vi "_Initialise Hardware Splash.vi"(8 "error in (no error)":errorcluster) -> (0 "error out":errorcluster, 2 "VISA Refnum out":refnum<visa-resource-name>, 3 "Enabled Hardware":T1)   [LabVIEW 2020]
uses:
  _Controls/Enabled Hardware.ctl
panel:
  in  "Enabled Hardware":T1=[{"Enable"=TRUE, "Status"=FALSE, "Device"="Confocal"}, {"Enable"=TRUE, "Status"=FALSE, "Device"="Pinhole"}, {"Enable"=TRUE, "Status"=FALSE, "Device"="Piezo"}, {"Enable"=TRUE, "Status"=FALSE, "Device"="iFlex"}, {"Enable"=TRUE, "Status"=FALSE, "Device"="Manlight"}, {"Enable"=TRUE, "Status"=FALSE, "Device"="SLM"}, {"Enable"=FALSE, "Status"=FALSE, "Device"="Camera"}]
  in  "Review":bool
  in  "Scan For Missing":bool
  out "SLM":bool
  out "iFlex":bool
  out "Manlight":bool
  out "Pinhole":bool
  out "PIFOC":bool
  out "Confocal":bool
  in  "animation":u16(ring)
  out "Status":string
  in  "Start":bool
  # "TweezerTron"
  # "Scanning for system hardware."
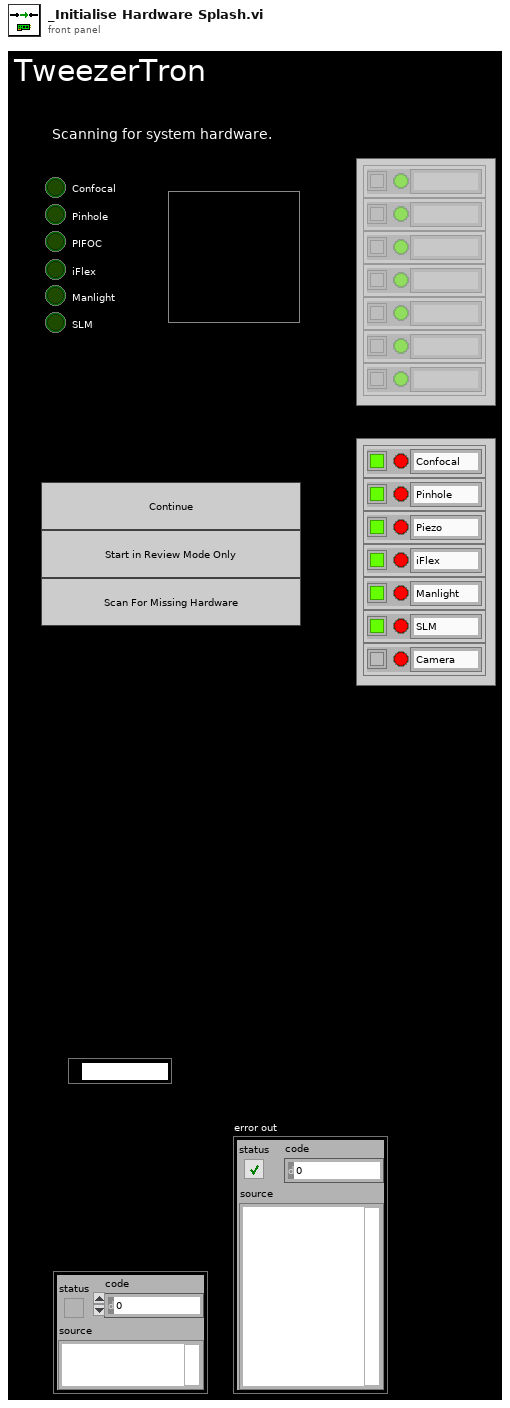
[diagram p1: front panel]
types:
  T1 = typedef "Enabled Hardware.ctl" = cluster{"Enable":bool, "Status":bool, "Device":string}[]
  T2 = typedef "Enabled Hardware.ctl" = cluster{"Confocal":cluster{"Enable":bool, "Status":bool}, "Pinhole":cluster{"Enable":bool, "Status":bool}, "Piezo":cluster{"Enable":bool, "Status":bool}, "iFlex":cluster{"Enable":bool, "Status":bool}, "SLM":cluster{"Enable":bool, "Status":bool}, "Manlight":cluster{"Enable":bool, "Status":bool}}
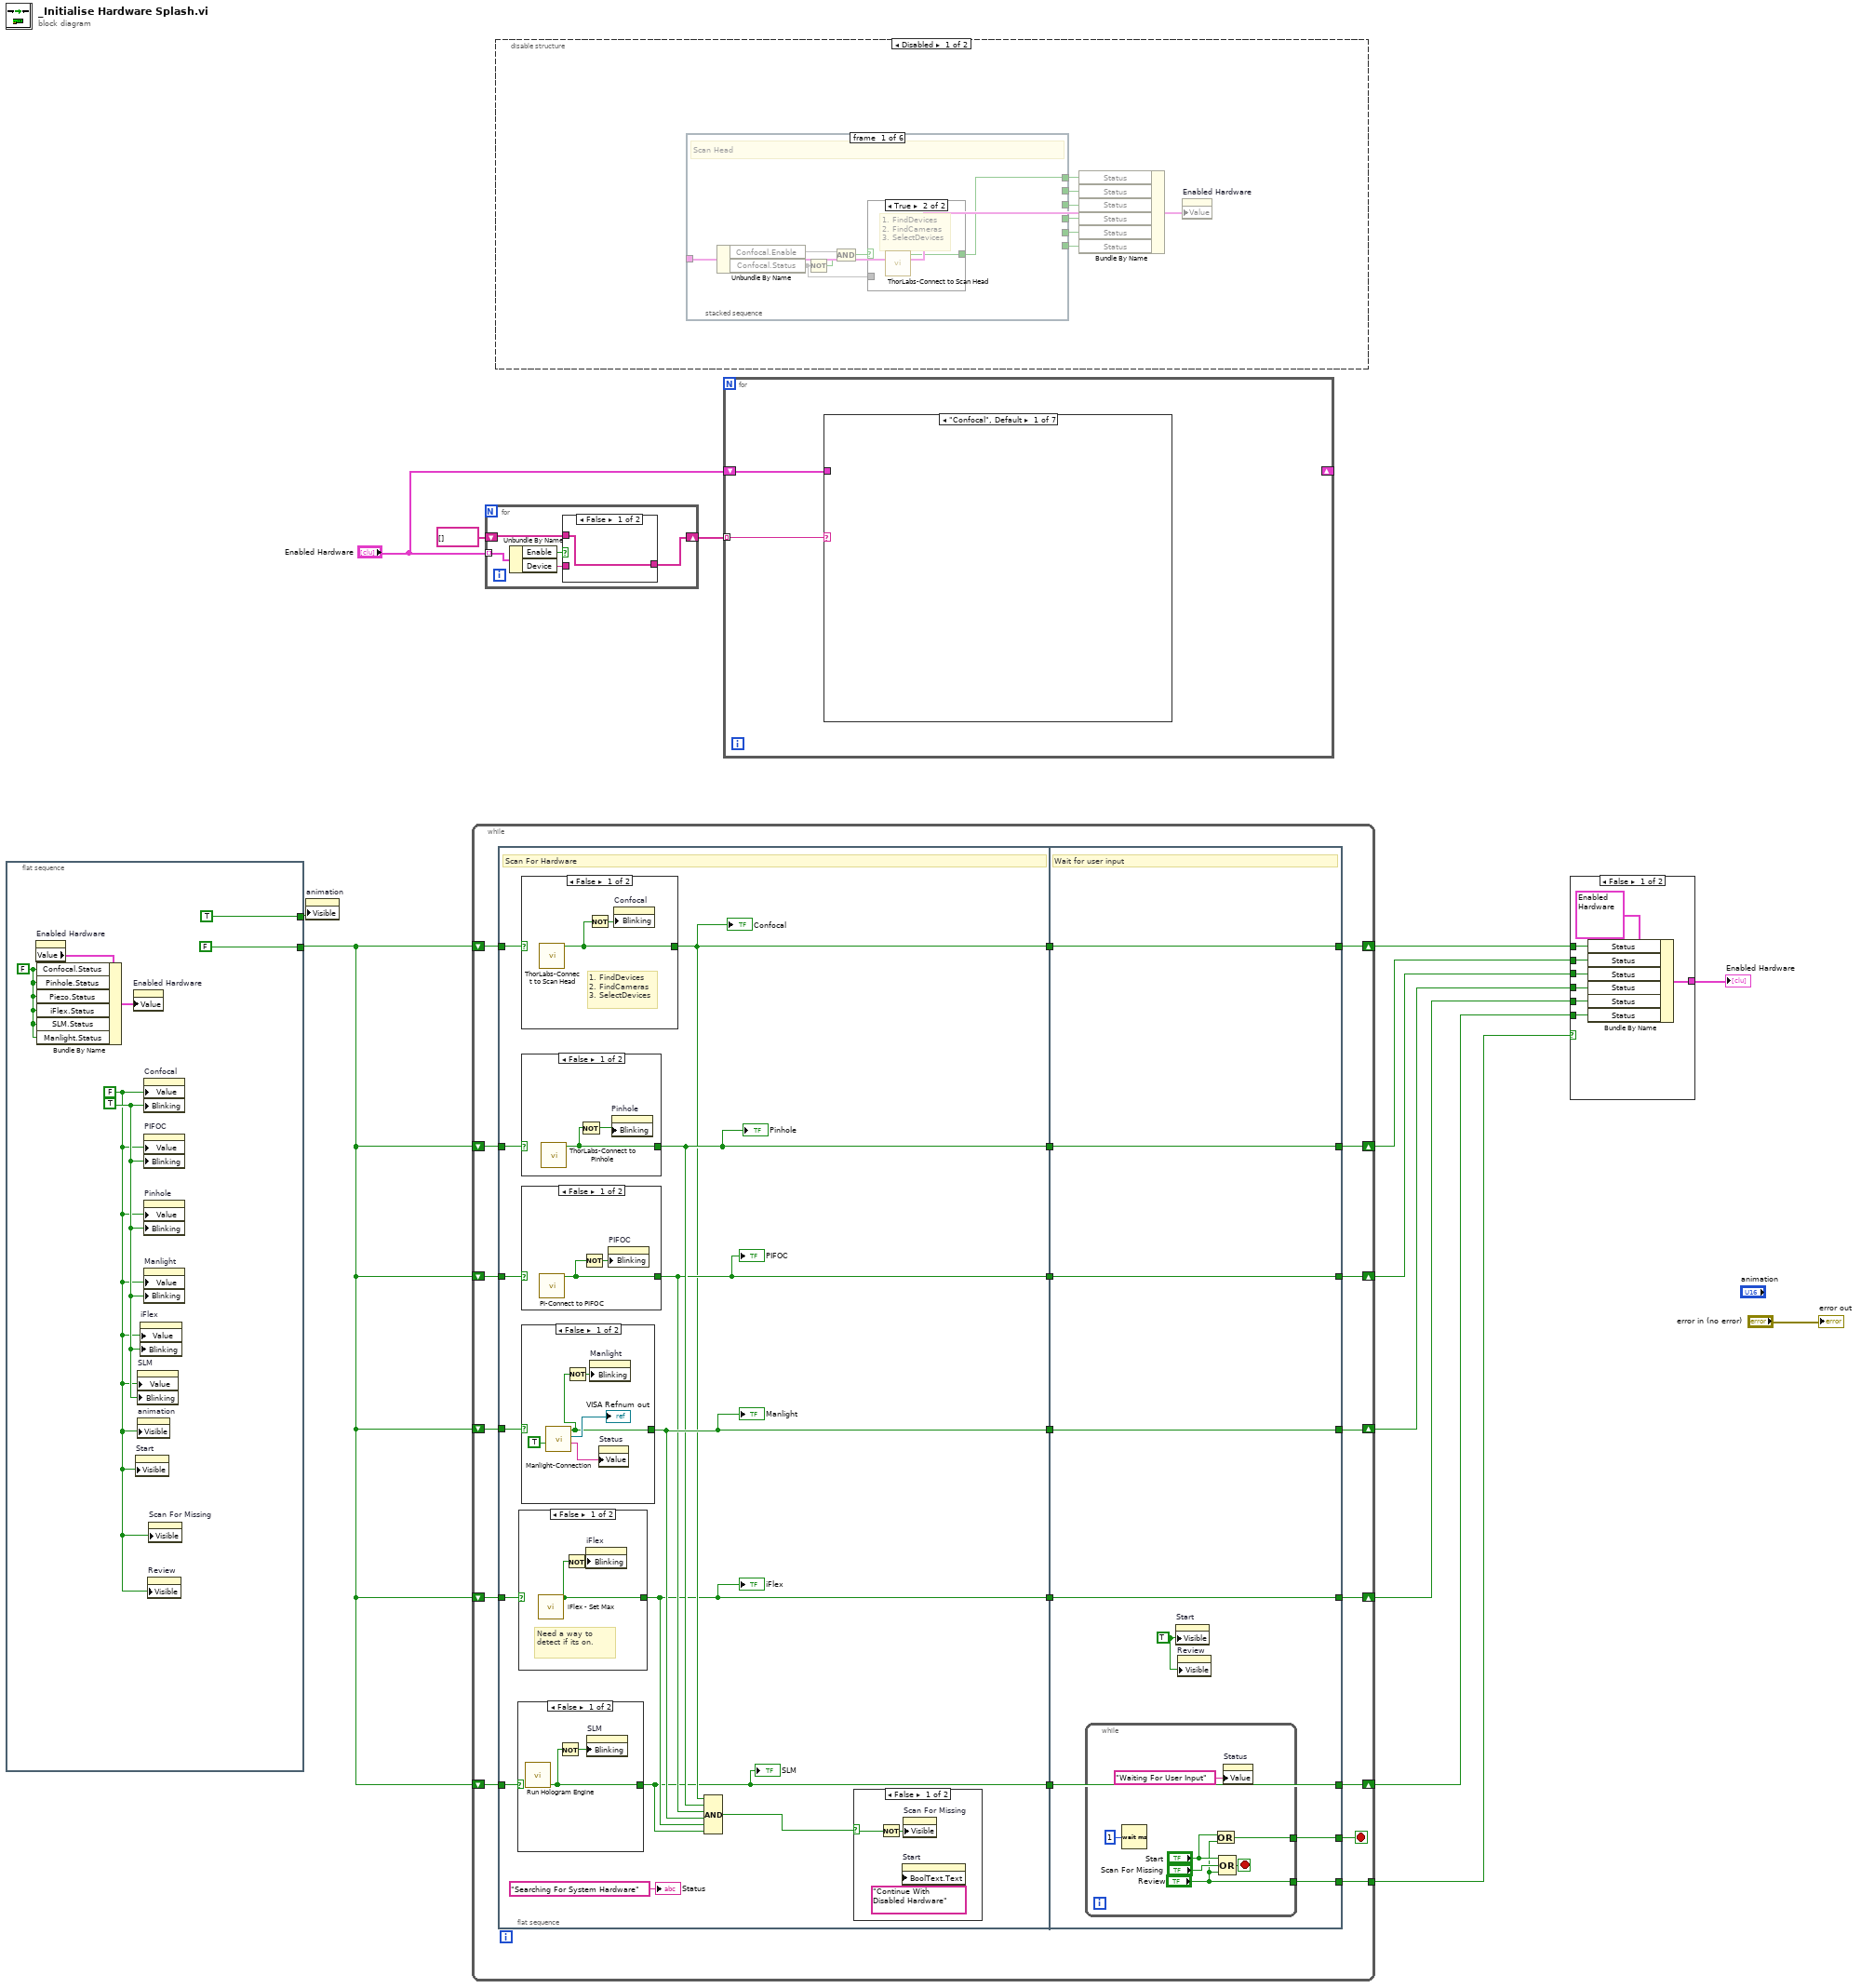
[diagram p0: block diagram]
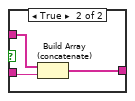
[diagram p2: hidden frame]
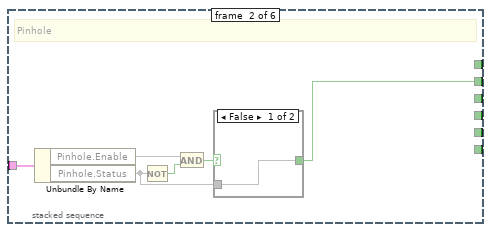
[diagram p10: hidden frame]
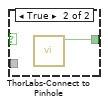
[diagram p11: hidden frame]
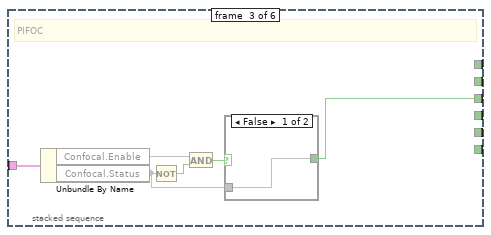
[diagram p12: hidden frame]
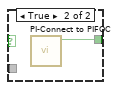
[diagram p13: hidden frame]
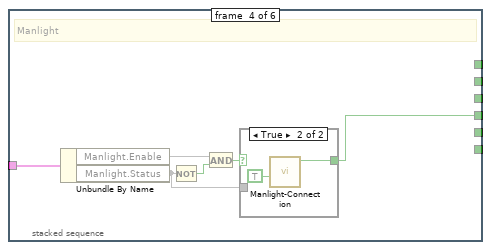
[diagram p14: hidden frame]
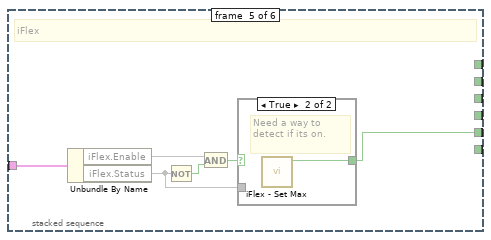
[diagram p16: hidden frame]
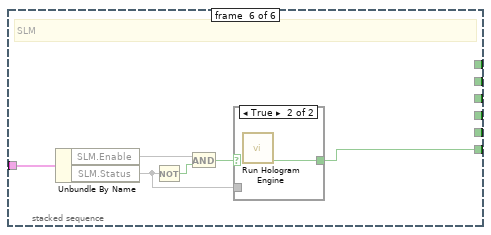
[diagram p18: hidden frame]
diagram:
  n1 = flat-sequence {
    tunnel: [FALSE] -> w6
    tunnel: [TRUE ("Visible")] -> w7
    frame #0 {
      w15 = FALSE ("Confocal.Status")
      w19 = TRUE
      w18 = FALSE ("Confocal")
      n2 = property on="Enabled Hardware" class="Arr (strict)"() -> ("Value"=w16:T2)  [unwired: 2 in, 2 out]
      n3 = Bundle By Name(cluster=w16, "Confocal.Status"=w15, "Pinhole.Status"=w15, "Piezo.Status"=w15, "iFlex.Status"=w15, "SLM.Status"=w15, "Manlight.Status"=w15) -> (w17:T2)
      n4 = property on="Enabled Hardware" class="Arr (strict)"("Value"=w17) -> ()  [unwired: 2 in, 2 out]
      n5 = property on="Start" class="Bool"("Visible"=w18) -> ()  [unwired: 2 in, 2 out]
      n6 = property on="SLM" class="Bool (strict)"("Value"=w18, "Blinking"=w19) -> ()  [unwired: 2 in, 2 out]
      n7 = property on="animation" class="Ring (strict)"("Visible"=w18) -> ()  [unwired: 2 in, 2 out]
      n8 = property on="iFlex" class="Bool (strict)"("Value"=w18, "Blinking"=w19) -> ()  [unwired: 2 in, 2 out]
      n9 = property on="Confocal" class="Bool (strict)"("Value"=w18, "Blinking"=w19) -> ()  [unwired: 2 in, 2 out]
      n10 = property on="PIFOC" class="Bool (strict)"("Value"=w18, "Blinking"=w19) -> ()  [unwired: 2 in, 2 out]
      n11 = property on="Pinhole" class="Bool (strict)"("Value"=w18, "Blinking"=w19) -> ()  [unwired: 2 in, 2 out]
      n12 = property on="Manlight" class="Bool (strict)"("Value"=w18, "Blinking"=w19) -> ()  [unwired: 2 in, 2 out]
      n13 = property on="Review" class="Bool"("Visible"=w18) -> ()  [unwired: 2 in, 2 out]
      n14 = property on="Scan For Missing" class="Bool"("Visible"=w18) -> ()  [unwired: 2 in, 2 out]
    }
  }
  n15 = property on="animation" class="Ring (strict)"("Visible"=w7) -> ()  [unwired: 2 in, 2 out]
  n16 = while {
    shift-right: [w34] -> w13
    shift-left: w6 -> [w41]
    shift-right: [w36] -> w12
    shift-left: w6 -> [w40]
    shift-right: [w35] -> w11
    shift-left: w6 -> [w39]
    shift-right: [w37] -> w10
    shift-left: w6 -> [w38]
    shift-right: [w32] -> w8
    shift-left: w6 -> [w33]
    shift-right: [w25] -> w5
    shift-left: w6 -> [w26]
    tunnel: [w22] -> w4
    stop <- w23 stop-if-true
    n17 = flat-sequence {
      tunnel: [w55] -> w31
      tunnel: [w54] -> w30
      tunnel: [w53] -> w29
      tunnel: [w52] -> w28
      tunnel: [w51] -> w27
      tunnel: [w50] -> w24
      tunnel: w26 -> [w43]
      tunnel: w33 -> [w44]
      tunnel: w38 -> [w45]
      tunnel: w39 -> [w46]
      tunnel: w40 -> [w47]
      tunnel: w41 -> [w48]
      tunnel: [w85] -> w32
      tunnel: [w86] -> w34
      tunnel: [w87] -> w35
      tunnel: [w88] -> w36
      tunnel: [w89] -> w37
      tunnel: w31 -> [w89]
      tunnel: w30 -> [w88]
      tunnel: w29 -> [w87]
      tunnel: w28 -> [w86]
      tunnel: w27 -> [w85]
      tunnel: [w84] -> w25
      tunnel: w24 -> [w84]
      tunnel: [w83] -> w23
      tunnel: [w82] -> w22
      frame #0 {
        # "Scan For Hardware"
        n18 = case shown="False" w43 {
          selector: w43 -> [_ w58]
          tunnel: [w56 w58] -> w50
          frame False {
            n19 = call "Run Hologram Engine.vi"() -> ("status"=w56:bool)  [unwired: 11 in]
            n20 = Not(x=w56) -> (.not. x?=w57:bool)
            n21 = property on="SLM" class="Bool (strict)"("Blinking"=w57) -> ()  [unwired: 2 in, 2 out]
          }
          frame True {
          }
        }
        "SLM" <- w50
        n22 = case shown="False" w44 {
          selector: w44 -> [_ w61]
          tunnel: [w59 w61] -> w51
          frame False {
            # "Need a way to detect if its on."
            n23 = call "iFlex - Set Max.vi"() -> ("iFlex Enabled"=w59:bool)  [unwired: 11 in]
            n24 = Not(x=w59) -> (.not. x?=w60:bool)
            n25 = property on="iFlex" class="Bool (strict)"("Blinking"=w60) -> ()  [unwired: 2 in, 2 out]
          }
          frame True {
          }
        }
        "iFlex" <- w51
        n26 = case shown="False" w48 {
          selector: w48 -> [_ w76]
          tunnel: [w74 w76] -> w52
          frame False {
            # "1. FindDevices\n2. FindCameras\n3. SelectDevices"
            n27 = call "ThorLabs-Connect to Scan Head.vi"() -> ("ThorLabs Scan Head Connected"=w74:bool)  [unwired: 10 in, 1 out]
            n28 = Not(x=w74) -> (.not. x?=w75:bool)
            n29 = property on="Confocal" class="Bool (strict)"("Blinking"=w75) -> ()  [unwired: 2 in, 2 out]
          }
          frame True {
          }
        }
        "Confocal" <- w52
        n30 = case shown="False" w47 {
          selector: w47 -> [_ w73]
          tunnel: [w71 w73] -> w54
          frame False {
            n31 = call "ThorLabs-Connect to Pinhole.vi"() -> ("Thorlabs Pinhole Connected"=w71:bool)  [unwired: 10 in, 1 out]
            n32 = Not(x=w71) -> (.not. x?=w72:bool)
            n33 = property on="Pinhole" class="Bool (strict)"("Blinking"=w72) -> ()  [unwired: 2 in, 2 out]
          }
          frame True {
          }
        }
        "Pinhole" <- w54
        n34 = case shown="False" w46 {
          selector: w46 -> [_ w70]
          tunnel: [w68 w70] -> w53
          frame False {
            n35 = call "PI-Connect to PIFOC.vi"() -> ("No Errors"=w68:bool)  [unwired: 5 in, 2 out]
            n36 = Not(x=w68) -> (.not. x?=w69:bool)
            n37 = property on="PIFOC" class="Bool (strict)"("Blinking"=w69) -> ()  [unwired: 2 in, 2 out]
          }
          frame True {
          }
        }
        "PIFOC" <- w53
        n38 = case shown="False" w45 {
          selector: w45 -> [_ w67]
          tunnel: [w62 w67] -> w55
          frame False {
            n39 = call "Manlight-Connection.vi"("Connect?"=TRUE ("Connect")) -> ("Status"=w64:string, "VISA Refnum out"=→"VISA Refnum out":refnum<visa-resource-name>, "Manlight Laser Connected"=w62:bool)  [unwired: 3 in, 1 out]
            n40 = Not(x=w62) -> (.not. x?=w63:bool)
            n41 = property on="Manlight" class="Bool (strict)"("Blinking"=w63) -> ()  [unwired: 2 in, 2 out]
            n42 = property on="Status" class="Str"("Value"=w64) -> ()  [unwired: 2 in, 2 out]
          }
          frame True {
          }
        }
        "Manlight" <- w55
        n43 = Compound Arithmetic op=AND(w52, w54, w53, w55, w51, w50) -> (w49:bool)
        n44 = case shown="False" w49 {
          selector: w49 -> [w78 _]
          frame False {
            n45 = Not(x=w78) -> (.not. x?=w77:bool)
            n46 = property on="Start" class="Bool"("BoolText.Text"="Continue With Disabled Hardware") -> ()  [unwired: 2 in, 2 out]
            n47 = property on="Scan For Missing" class="Bool"("Visible"=w77) -> ()  [unwired: 2 in, 2 out]
          }
          frame True {
            n48 = property on="Start" class="Bool"("BoolText.Text"="Continue" ("Boolean Text.Text")) -> ()  [unwired: 2 in, 2 out]
          }
        }
        "Status" <- "Searching For System Hardware" ("string")
      }
      frame #1 {
        w81 = TRUE ("Visible")
        # "Wait for user input"
        n49 = while {
          tunnel: [w92] -> w83
          tunnel: ["Review"] -> w82
          stop <- w94 stop-if-true
          n50 = Wait (ms)(milliseconds to wait=u32 1) -> ()  [unwired: 1 out]
          n51 = Or(x="Start", y="Review") -> (x .or. y?=w92:bool)
          n52 = Compound Arithmetic op=OR("Start", "Scan For Missing", "Review") -> (w94:bool)
          n53 = property on="Status" class="Str"("Value"="Waiting For User Input" ("Status")) -> ()  [unwired: 2 in, 2 out]
        }
        n54 = property on="Start" class="Bool"("Visible"=w81) -> ()  [unwired: 2 in, 2 out]
        n55 = property on="Review" class="Bool"("Visible"=w81) -> ()  [unwired: 2 in, 2 out]
      }
    }
  }
  n56 = for {
    tunnel: "Enabled Hardware" -> [w101] mode=indexing
    shift-right: [w97] -> w1
    shift-left: string[] [] -> [w98]
    n57 = Unbundle By Name(w101) -> ("Enable"=w100:bool, "Device"=w99:string)
    n58 = case shown="False" w100 {
      tunnel: w99 -> [_ w105]
      tunnel: w98 -> [w102 w104]
      tunnel: [w102 w103] -> w97
      frame False {
      }
      frame True {
        n59 = Build Array (concatenate)(w104, w105) -> (w103:string[])
      }
    }
  }
  n60 = disable-structure shown="Disabled" {
    frame Disabled {
      n61 = stacked-sequence {
        tunnel: w112 -> [w119 w124 w133 w141 w150 w158]
        tunnel: [w115 _ _ _ _ _] -> w111
        tunnel: [_ w127 _ _ _ _] -> w110
        tunnel: [_ _ w131 _ _ _] -> w109
        tunnel: [_ _ _ w138 _ _] -> w108
        tunnel: [_ _ _ _ w148 _] -> w107
        tunnel: [_ _ _ _ _ w156] -> w106
        frame #0 {
          # "Scan Head"
          n62 = Unbundle By Name(w119) -> ("Confocal.Enable"=w116, "Confocal.Status"=w114)
          n63 = Not(x=w114) -> (.not. x?=w117:bool)
          n64 = And(x=w116, y=w117) -> (x .and. y?=w118:bool)
          n65 = case shown="True" w118 {
            tunnel: [w120 w121] -> w115
            tunnel: w114 -> [w120 _]
            frame False {
            }
            frame True {
              # "1. FindDevices\n2. FindCameras\n3. SelectDevices"
              n66 = call "ThorLabs-Connect to Scan Head.vi"() -> ("ThorLabs Scan Head Connected"=w121:bool)  [unwired: 10 in, 1 out]
            }
          }
        }
        frame #1 {
          # "Pinhole"
          n67 = Unbundle By Name(w124) -> ("Pinhole.Enable"=w125, "Pinhole.Status"=w122)
          n68 = Not(x=w122) -> (.not. x?=w126:bool)
          n69 = And(x=w125, y=w126) -> (x .and. y?=w123:bool)
          n70 = case shown="False" w123 {
            tunnel: [w128 w129] -> w127
            tunnel: w122 -> [w128 _]
            frame False {
            }
            frame True {
              n71 = call "ThorLabs-Connect to Pinhole.vi"() -> ("Thorlabs Pinhole Connected"=w129:bool)  [unwired: 10 in, 1 out]
            }
          }
        }
        frame #2 {
          # "PIFOC"
          n72 = Unbundle By Name(w133) -> ("Confocal.Enable"=w134, "Confocal.Status"=w130)
          n73 = Not(x=w130) -> (.not. x?=w135:bool)
          n74 = And(x=w134, y=w135) -> (x .and. y?=w132:bool)
          n75 = case shown="False" w132 {
            tunnel: [w136 w137] -> w131
            tunnel: w130 -> [w136 _]
            frame False {
            }
            frame True {
              n76 = call "PI-Connect to PIFOC.vi"() -> ("No Errors"=w137:bool)  [unwired: 5 in, 2 out]
            }
          }
        }
        frame #3 {
          # "Manlight"
          n77 = Unbundle By Name(w141) -> ("Manlight.Enable"=w142, "Manlight.Status"=w139)
          n78 = Not(x=w139) -> (.not. x?=w143:bool)
          n79 = And(x=w142, y=w143) -> (x .and. y?=w140:bool)
          n80 = case shown="True" w140 {
            tunnel: [w144 w145] -> w138
            tunnel: w139 -> [w144 _]
            frame False {
            }
            frame True {
              n81 = call "Manlight-Connection.vi"("Connect?"=TRUE ("Connect")) -> ("Manlight Laser Connected"=w145:bool)  [unwired: 3 in, 3 out]
            }
          }
        }
        frame #4 {
          # "iFlex"
          n82 = Unbundle By Name(w150) -> ("iFlex.Enable"=w151, "iFlex.Status"=w147)
          n83 = Not(x=w147) -> (.not. x?=w152:bool)
          n84 = And(x=w151, y=w152) -> (x .and. y?=w149:bool)
          n85 = case shown="True" w149 {
            tunnel: [w153 w154] -> w148
            tunnel: w147 -> [w153 _]
            frame False {
            }
            frame True {
              # "Need a way to detect if its on."
              n86 = call "iFlex - Set Max.vi"() -> ("iFlex Enabled"=w154:bool)  [unwired: 11 in]
            }
          }
        }
        frame #5 {
          # "SLM"
          n87 = Unbundle By Name(w158) -> ("SLM.Enable"=w160, "SLM.Status"=w155)
          n88 = Not(x=w155) -> (.not. x?=w159:bool)
          n89 = And(x=w160, y=w159) -> (x .and. y?=w157:bool)
          n90 = case shown="True" w157 {
            tunnel: [w161 w162] -> w156
            tunnel: w155 -> [w161 _]
            frame False {
            }
            frame True {
              n91 = call "Run Hologram Engine.vi"() -> ("status"=w162:bool)  [unwired: 11 in]
            }
          }
        }
      }
      n92 = Bundle By Name("Status"=w111, "Status"=w110, "Status"=w109, "Status"=w108, "Status"=w107, "Status"=w106) -> (w113:cluster{}, w112:cluster{})
      n93 = property on="Enabled Hardware" class="Arr (strict)"("Value"=w113) -> ()  [unwired: 2 in, 2 out]
    }
    frame Enabled {
    }
  }
  n94 = for {
    tunnel: w1 -> [w164] mode=indexing
    shift-right: _ -> [_]
    shift-left: "Enabled Hardware" -> [w163]
    n95 = case shown="\"Confocal\", Default" w164 {
      tunnel: w163 -> [_ _ _ _ _ _ _]
      frame "Confocal", Default {
      }
      frame "Pinhole" {
      }
      frame "Piezo" {
      }
      frame "iFlex" {
      }
      frame "Manlight" {
      }
      frame "SLM" {
      }
      frame "Camera" {
      }
    }
  }
  n96 = case shown="False" w4 {
    tunnel: w13 -> [w172 _]
    tunnel: w12 -> [w171 _]
    tunnel: w11 -> [w170 _]
    tunnel: w10 -> [w169 _]
    tunnel: [w168 T2 {"Confocal"={"Enable"=FALSE, "Status"=FALSE}, "Pinhole"={"Enable"=FALSE, "Status"=FALSE}, "Piezo"={"Enable"=FALSE, "Status"=FALSE}, "iFlex"={"Enable"=FALSE, "Status"=FALSE}, "SLM"={"Enable"=FALSE, "Status"=FALSE}, "Manlight"={"Enable"=FALSE, "Status"=FALSE}} ("Enabled Hardware")] -> w9
    tunnel: w8 -> [w167 _]
    tunnel: w5 -> [w166 _]
    frame False {
      n97 = Bundle By Name(cluster=T1 [{"Enable"=TRUE, "Status"=FALSE, "Device"="Confocal"}, {"Enable"=TRUE, "Status"=FALSE, "Device"="Pinhole"}, {"Enable"=TRUE, "Status"=FALSE, "Device"="Piezo"}, {"Enable"=TRUE, "Status"=FALSE, "Device"="iFlex"}, {"Enable"=TRUE, "Status"=FALSE, "Device"="Manlight"}, {"Enable"=TRUE, "Status"=FALSE, "Device"="SLM"}, {"Enable"=FALSE, "Status"=FALSE, "Device"="Camera"}] ("Enabled Hardware"), "Status"=w172, "Status"=w171, "Status"=w170, "Status"=w169, "Status"=w167, "Status"=w166) -> (w168:cluster{})
    }
    frame True {
    }
  }
  "Enabled Hardware" <- w9
  "error out" <- "error in (no error)"
